vi "Write Active Plot.vi"(8 "error in (no error)":errorcluster, 10 "ActPlot":u32, 11 "WaveformChart.lvclass in":refnum<class "WaveformChart.lvclass">) -> (0 "error out":errorcluster, 3 "WaveformChart.lvclass out":refnum<class "WaveformChart.lvclass">)   [LabVIEW 2015, in "WaveformChart.lvclass"]
uses:
  WaveformChart.lvclass
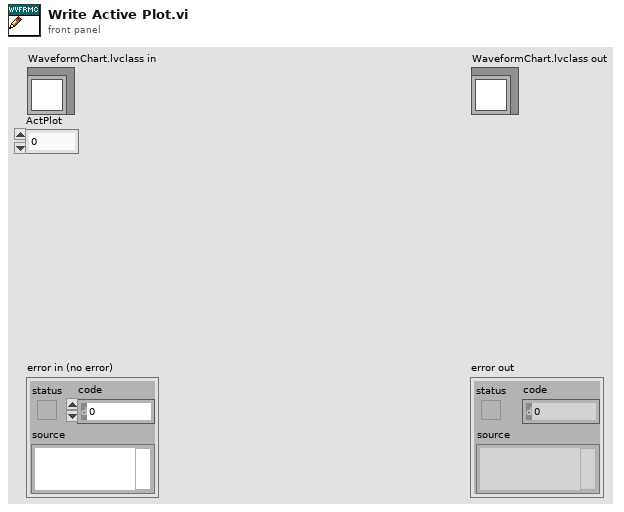
[diagram p1: front panel]
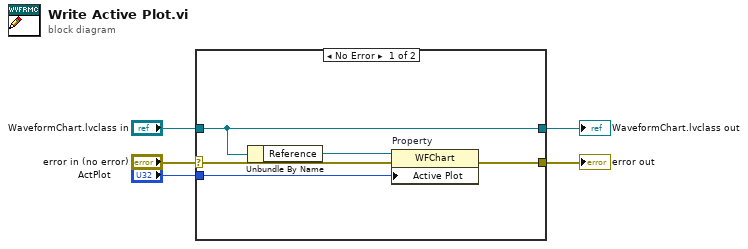
[diagram p0: block diagram]
diagram:
  n1 = case shown="No Error" "error in (no error)" {
    selector: "error in (no error)" -> [w6 w12]
    tunnel: [w10 w12] -> w4
    tunnel: [w8 w11] -> w2
    tunnel: "WaveformChart.lvclass in" -> [w8 w11]
    tunnel: "ActPlot" -> [w9 _]
    frame No Error {
      n2 = Unbundle By Name(w8) -> ("Reference"=w7:refnum<vi>)
      n3 = property on="Property" class="WFChart"(reference=w7, error in=w6, "Active Plot"=w9) -> (error out=w10:errorcluster)  [unwired: 1 out]
    }
    frame Error {
    }
  }
  "error out" <- w4
  "WaveformChart.lvclass out" <- w2
